vi "_CSM Message Communication Panel.vi"() -> ()   [LabVIEW 2017]
uses:
  _Support/Typedef/_CSM_GlobalLog_MSG.ctl
  _Support/Typedef/_CSM_Response Source Message.ctl
  _Support/Typedef/_CSM_GlobalLog_MSG_TYPE.ctl
  _Support/Priority Queue/Priority Queue.lvclass/Priority Queue.ctl
  _Polymophic/Add State(s) to Queue By BOOL(Element).vi
  _Polymophic/Build Synchronous Message with Arguments.vi
  _Polymophic/Build No-Reply Asynchronous Message with Arguments.vi
  AdvanceAPI/CSM - Keywords.vi
  AdvanceAPI/CSM - Convert Error to Argument.vi
  <vilib>/Utility/error.llb/Clear Errors.vi
  _Support/GlobalEvent/Gevt-ThreadQueueName.vi
  _Support/Common/Trim Single line Text.vi
  _Support/Process/CSMP-Sync Call.vi
  Utility/uuid.vi
  Utility/Build Error Cluster.vi
  Utility/Trim Both Whitespace.vi
  _Support/Process/CSMP-Async Call.vi
  _Support/CSMQ/_CSMObj-Message Check.vi
  _Support/CSMQ/_CSMObj-Enqueue Cross-Module Message.vi
  _Support/CSMQ/_CSMOFGV Get.vi
  _Support/Priority Queue/Enqueue Element.vi
  _Support/GlobalEvent/FGV-GlobalEventRef.vi
  <vilib>/Utility/config.llb/Read Key (String).vi
  <vilib>/Utility/config.llb/Write Key (String).vi
  _Support/FGV-BroadcastRegistry/global-CSMQ FGV Change Flag.vi
  _Support/CSMQ/_CSMOFGV.vi
  _Support/Error/CSM No Target Error.vi
  _Support/Error/CSM Not Allowed Message.vi
  _Support/Error/CSM Target Error.vi
  _Support/Error/CSM Unhandled State Error.vi
  _Support/Error/CSM Target Timeout Error.vi
  _Support/Message/Parse State with Arguments String.vi
  Communicable State Machine.lvlib
  <vilib>/Utility/config.llb/NI_LVConfig.lvlib
panel:
  in  "History":i32(listbox)
  in  "CSM 2":string(combo)
  in  "Refresh":bool
  in  "Arguments":string
  out "Response":string
  in  "Clear History":bool
  in  "History Length":i32=50 min=20 max=1000 step=1
  in  "CSM":string(combo)
  in  "Refresh CSM":bool
  in  "RespTMO(ms)":i32=10000 format="%.0p"
  in  "Sync (-@) 2":bool
  in  "Sync (-@)":bool
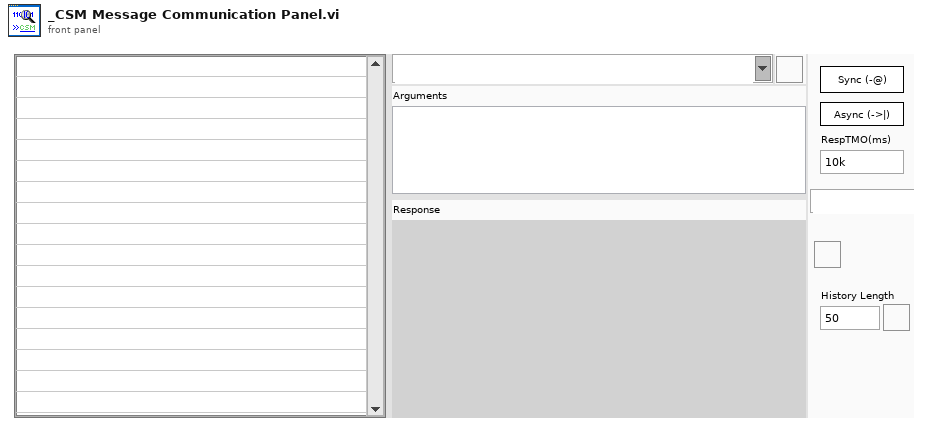
[diagram p1: front panel]
types:
  T1 = enum32{"Invalid", "Standard", "Closed", "Hidden", "Minimized", "Maximized"}
  T2 = enum32{"invalid app kind", "Development System", "Run Time System", "Student Edition", "Embedded LabVIEW", "Evaluation", "Custom"}
  T3 = cluster{"Shift":bool, "Ctrl":bool, "Alt":bool, "Cmd":bool, "Opt":bool}
  T4 = cluster{"Core":cluster{"Current VI Reference":refnum<vi>, "Close Panel on Exit?":bool}, "CSM Global Log Event":refnum<user-event>, "lvlps File":path, "MessageList":string[], "Toobar.advance":refnum<vi>[]}
  T5 = typedef "LVPoint32TypeDef.ctl" = cluster{"Horizontal":i32, "Vertical":i32}
  T6 = cluster{"Current VI Reference":refnum<vi>, "Close Panel on Exit?":bool}
  T7 = typedef "NI_LVConfig.lvlib/Config Data RefNum.ctl" = refnum<k1>
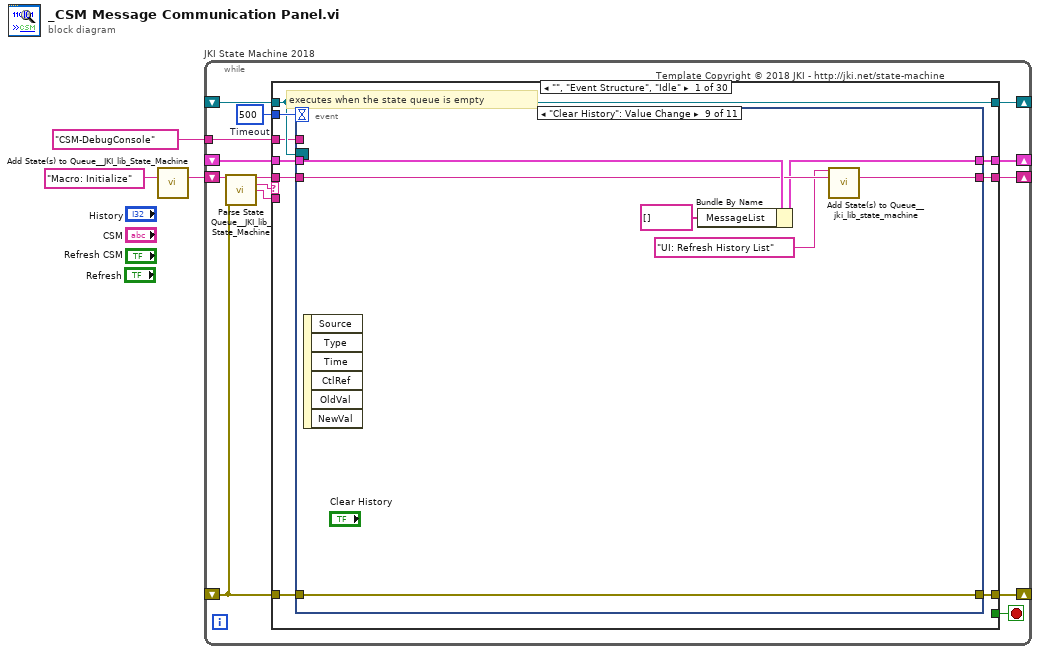
[diagram p0: block diagram]
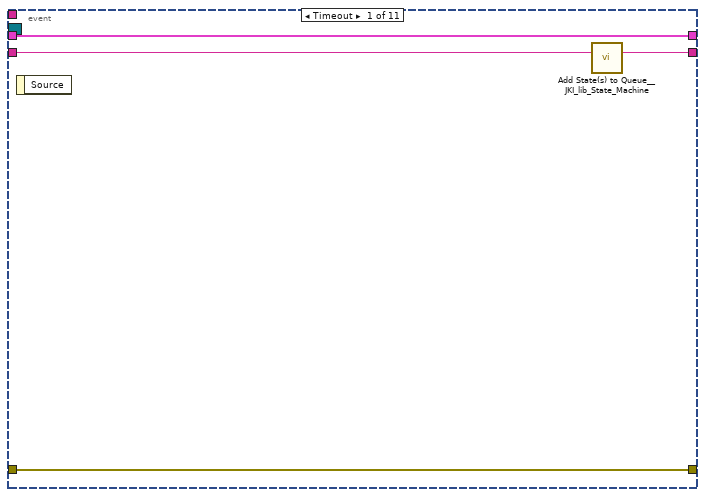
[diagram p2: hidden frame]
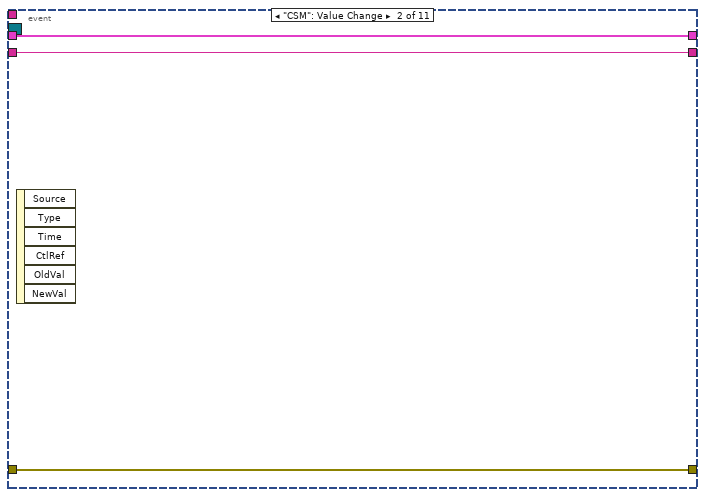
[diagram p3: hidden frame]
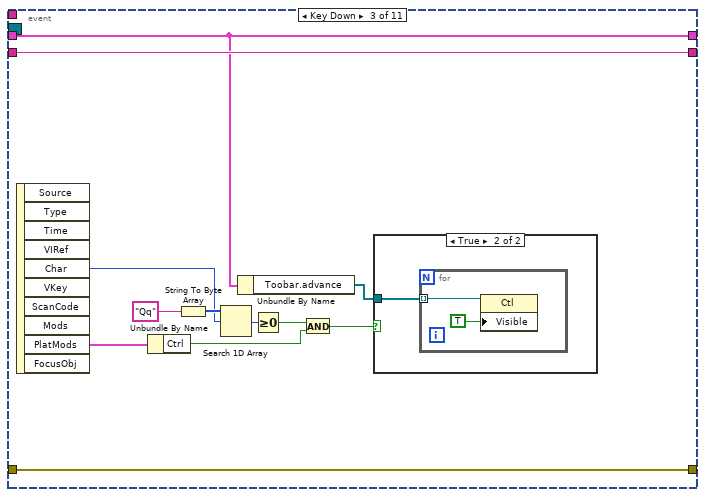
[diagram p4: hidden frame]
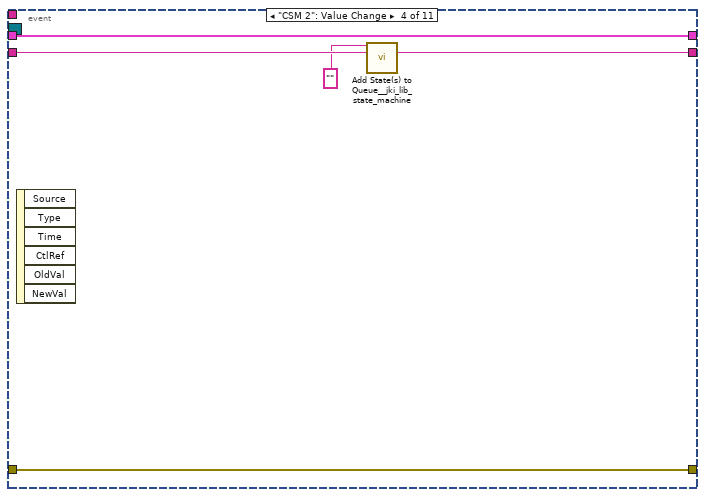
[diagram p6: hidden frame]
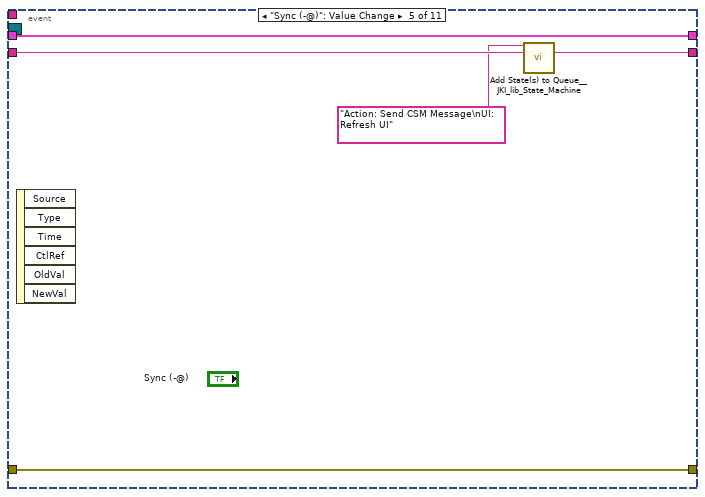
[diagram p7: hidden frame]
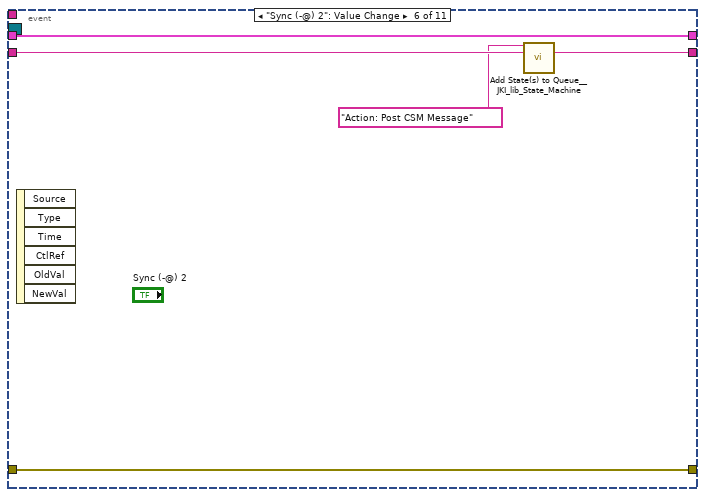
[diagram p8: hidden frame]
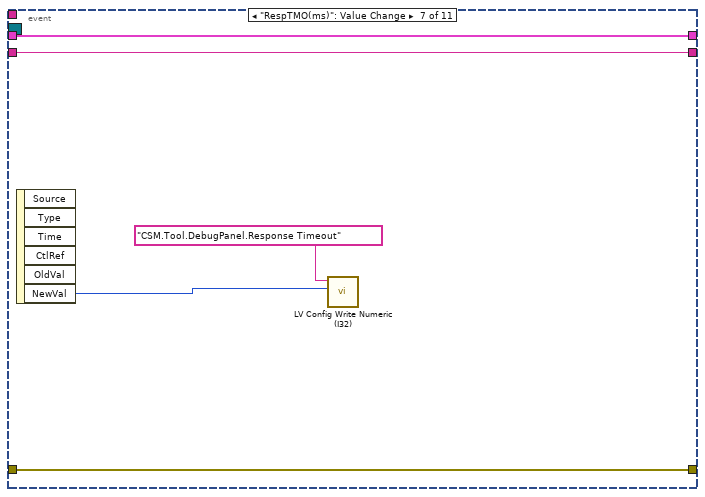
[diagram p9: hidden frame]
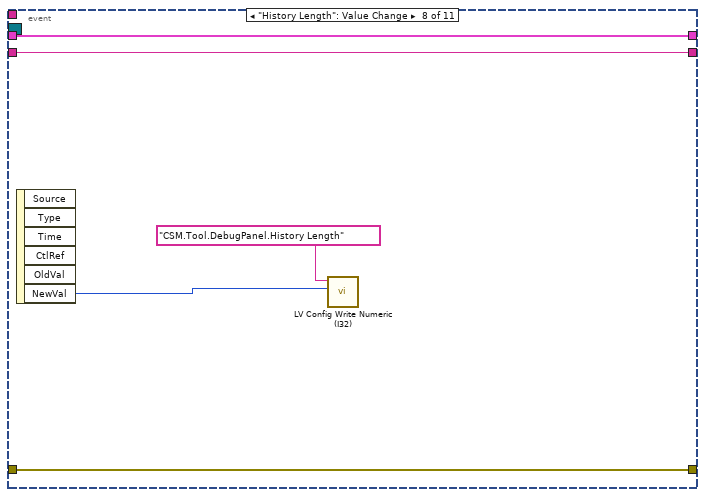
[diagram p10: hidden frame]
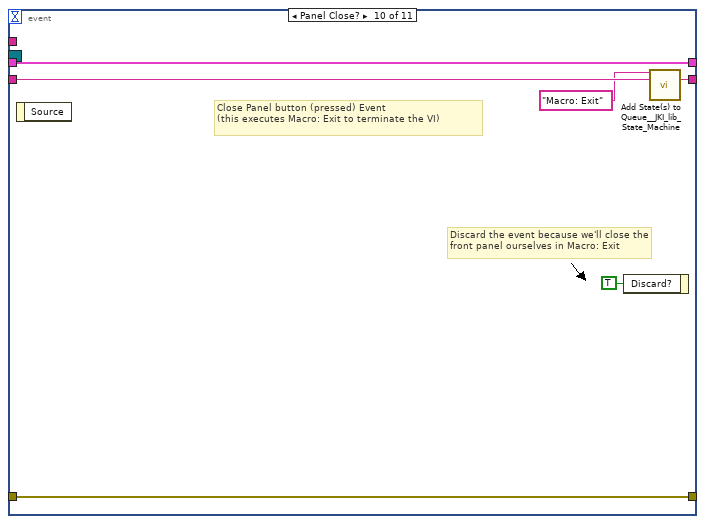
[diagram p11: hidden frame]
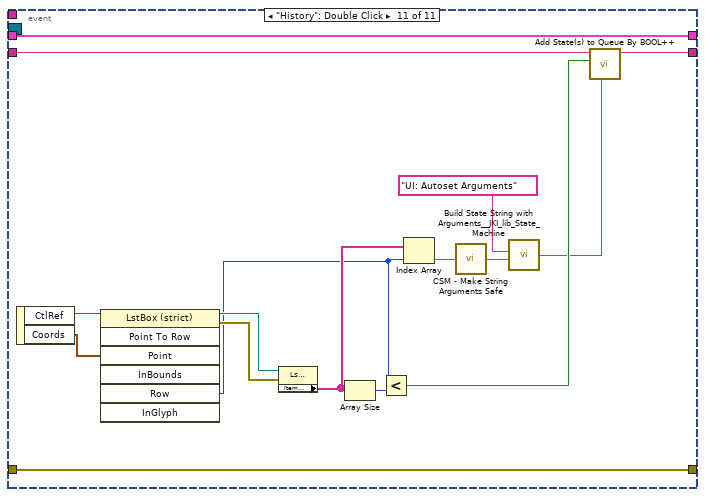
[diagram p12: hidden frame]
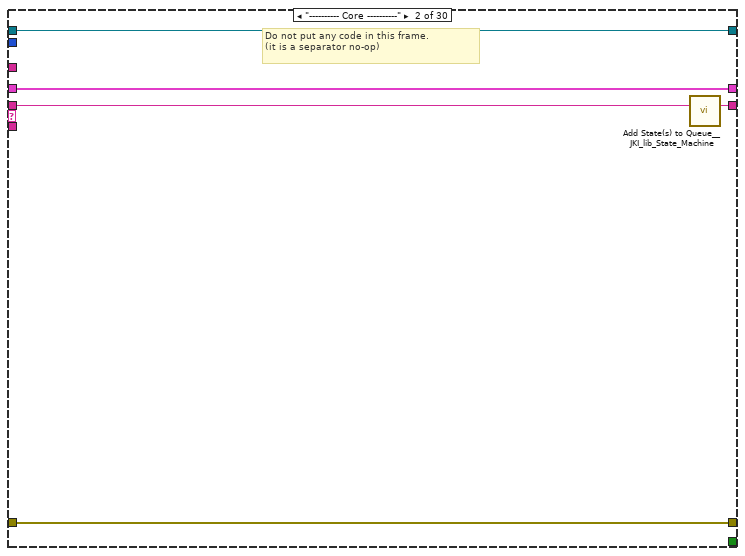
[diagram p13: hidden frame]
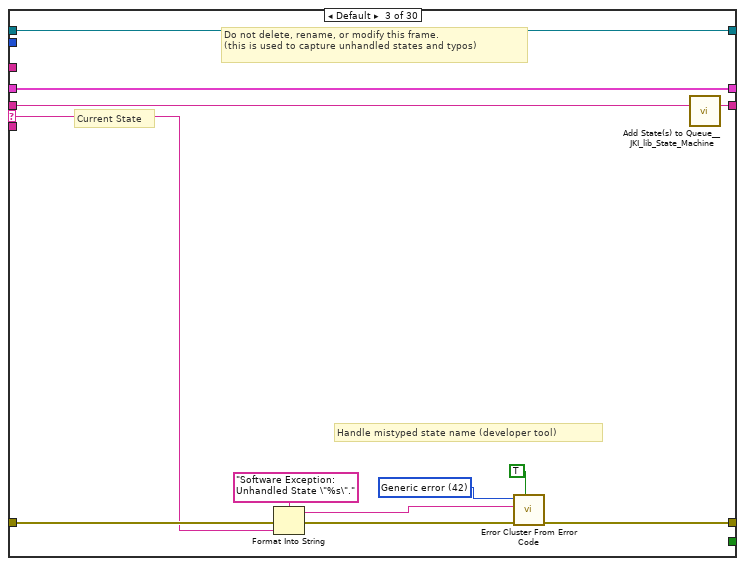
[diagram p14: hidden frame]
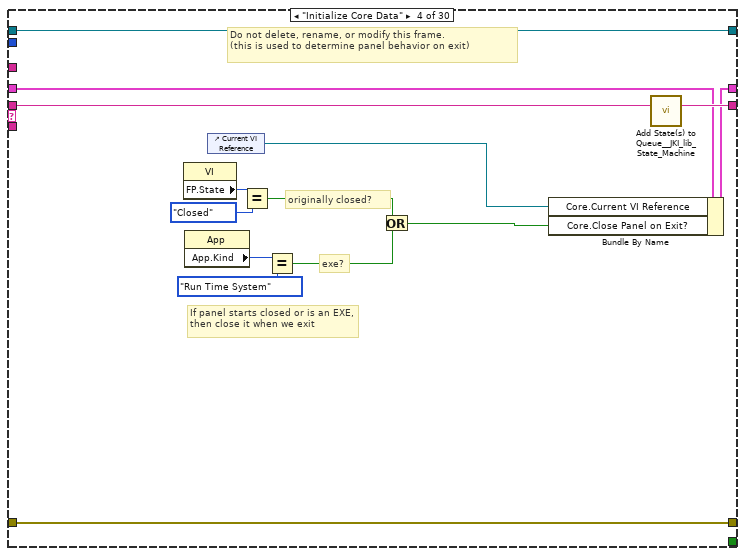
[diagram p15: hidden frame]
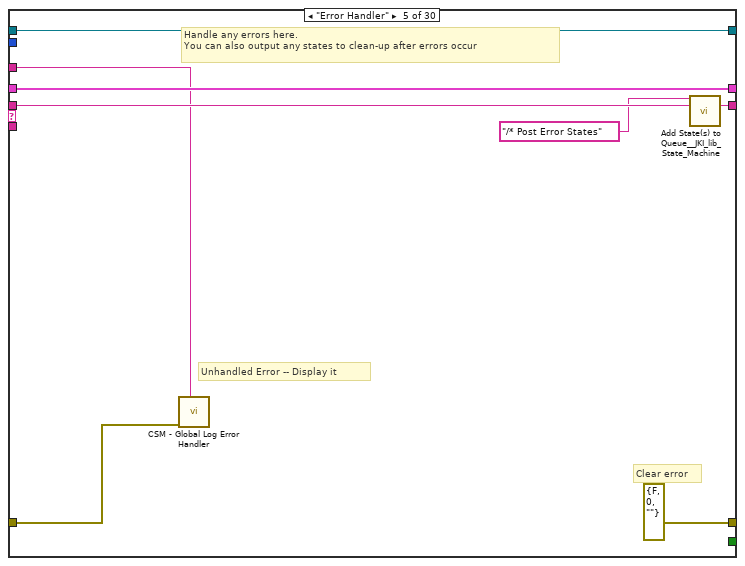
[diagram p16: hidden frame]
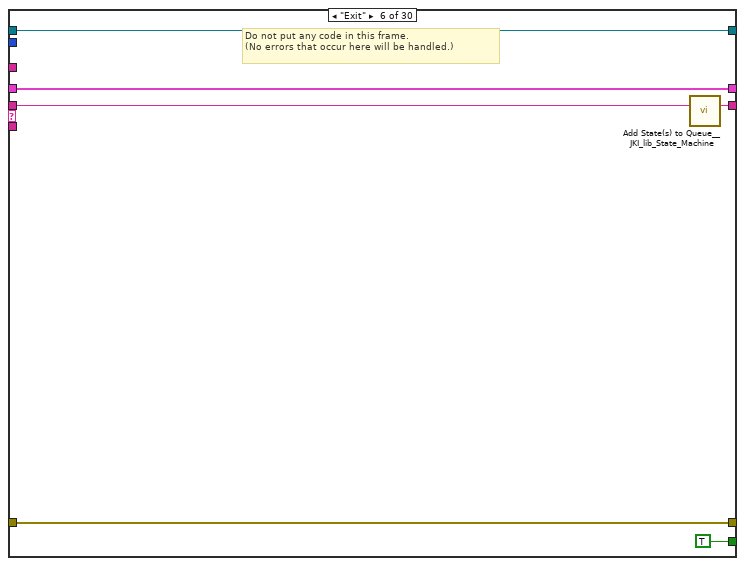
[diagram p17: hidden frame]
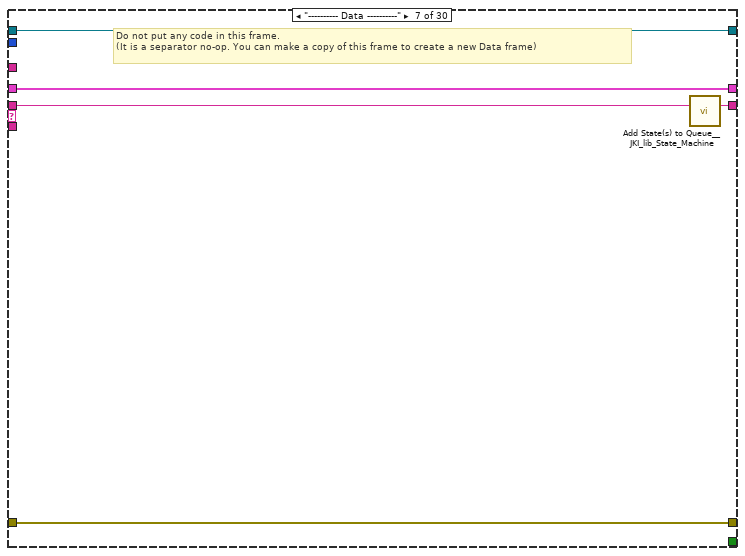
[diagram p18: hidden frame]
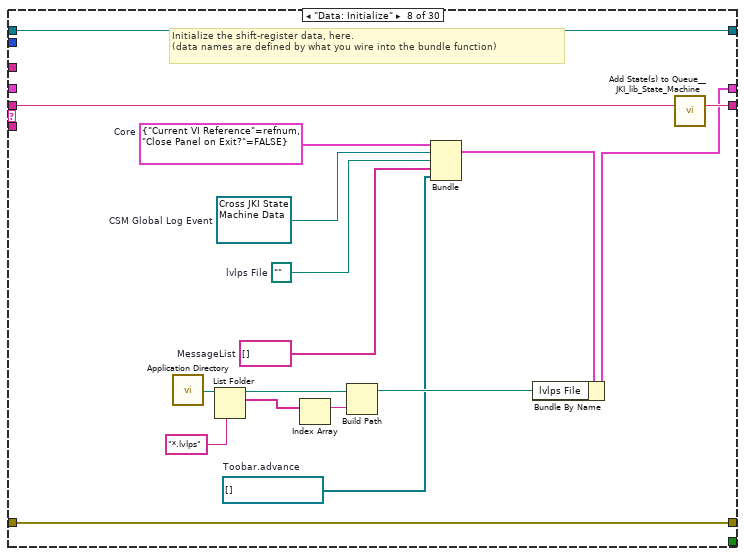
[diagram p19: hidden frame]
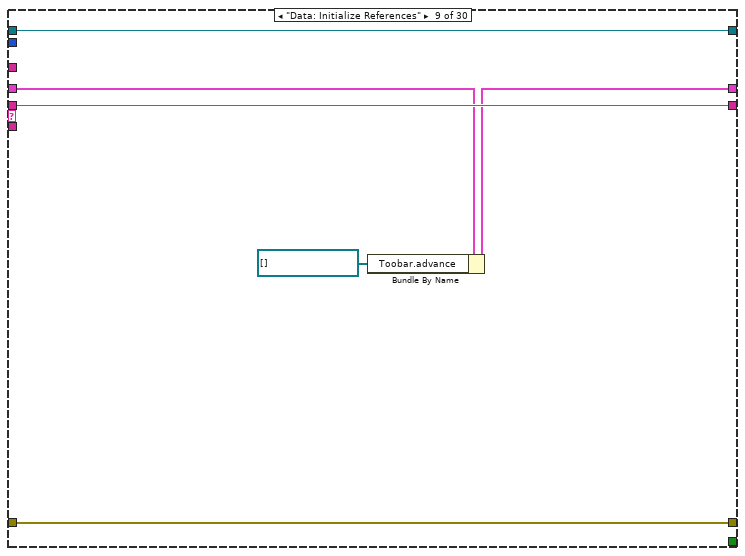
[diagram p20: hidden frame]
diagram:
  n1 = call <vilib>:"Add State(s) to Queue__JKI_lib_State_Machine.vi"("State(s) in (\"\")"="Macro: Initialize") -> ("States Out"=w2:string)  [unwired: 14 in]
  n2 = while "JKI State Machine 2018" {
    shift-right: [w10] -> _
    shift-left: _ -> [w9]
    shift-right: [w13] -> _
    shift-left: _ -> [w7]
    shift-right: [w12] -> _
    shift-left: w2 -> [w14]
    shift-right: [w6] -> _
    shift-left: _ -> [w5]
    tunnel: "CSM-DebugConsole" -> [w4]
    stop <- w11 stop-if-true
    w8 = 500  # Timeout
    # "Template Copyright © 2018 JKI - http://jki.net/state-machine"
    n3 = call <vilib>:"Parse State Queue__JKI_lib_State_Machine.vi"("State Queue"=w14, "Error In (no error)"=w7) -> ("Remaining States"=w16:string, "Current State"=w17:string, "Arguments"=w15:string)  [unwired: 11 in]
    n4 = case shown="\"\", \"Event Structure\", \"Idle\"" w17 {
      selector: w17 -> [_ _ w109 _ _ _ _ _ _ _ _ _ _ _ _ _ _ _ _ _ _ _ _ _ _ _ _ _ _ _]
      tunnel: w16 -> [w26 w107 w113 w133 w141 w147 w152 w169 w174 w186 w217 w248 w264 w269 w276 w283 w288 w300 w310 w322 w401 w412 w425 w429 w435 w441 w452 w457 w467 w489]
      tunnel: w15 -> [_ _ _ _ _ _ _ _ _ _ _ w243 _ _ _ _ _ _ w305 w316 w399 _ _ _ _ _ _ _ _ _]
      tunnel: w9 -> [w24 w104 w111 w126 w138 w145 w149 _ w173 w179 w210 w245 w259 w266 w274 w279 w285 w296 w308 w318 w396 w410 w424 w427 w432 w438 w449 w454 w465 w487]
      tunnel: [w23 w105 w115 w130 errorcluster {"status"=FALSE, "code"=0, "source"=""} ("error out") w144 w150 w166 w175 w178 w211 w246 w260 w267 w272 w280 w286 w298 w306 w319 w402 w413 w426 w430 w433 w439 w450 w455 w461 w485] -> w13
      tunnel: w7 -> [w22 w105 w114 w130 w137 w144 w150 w166 w175 _ _ w246 w261 w267 _ _ w286 w298 w307 w320 w402 w413 w426 w430 w433 w439 w450 w455 _ _]
      tunnel: [w25 w106 w112 w132 w140 w146 w151 w168 w174 w186 w217 w248 w263 w268 w275 w282 w287 w299 w309 w321 w401 w412 w425 w429 w434 w440 w451 w456 w466 w488] -> w12
      tunnel: [_ _ _ _ _ TRUE _ _ _ _ _ _ _ _ _ _ _ _ _ _ _ _ _ _ _ _ _ _ _ _] -> w11
      tunnel: [w21 w104 w111 w131 w138 w145 w149 w161 w171 w184 w210 w239 w259 w266 w274 w279 w285 w296 w308 w318 w396 w410 w424 w427 w432 w438 w449 w454 w465 w487] -> w10
      tunnel: w8 -> [w20 _ _ _ _ _ _ _ _ _ _ _ _ _ _ _ _ _ _ _ _ _ _ _ _ _ _ _ _ _]
      tunnel: [w19 w103 w108 w120 w135 w142 w148 w164 w172 w185 w216 w247 w258 w265 w273 w281 w284 w297 w304 w315 w400 w411 w423 w428 w431 w436 w442 w453 w464 w486] -> w6
      tunnel: w5 -> [w19 w103 w108 w120 w135 w142 w148 w164 w172 w185 w216 w247 w258 w265 _ w281 w284 w297 w304 w315 w400 w411 w423 w428 w431 w436 w442 w453 w464 w486]
      tunnel: w4 -> [w18 _ _ _ w134 _ _ _ _ w176 w208 _ _ _ _ _ _ _ _ _ _ _ _ _ _ _ _ _ _ _]
      frame "", "Event Structure", "Idle" {
        # "executes when the state queue is empty"
        n5 = event shown="[8] \"Clear History\": Value Change" {
          selector: w19 -> [_ _ _ _ _ _ _ _ _ _ _]
          dyn-events: _ -> [_ _ _ _ _ _ _ _ _ _ _]
          timeout: w20 -> [_ _ _ _ _ _ _ _ _ _ _]
          tunnel: w26 -> [w30 w33 w45 w50 w55 w60 w68 w73 w77 w86 w94]
          tunnel: [w29 w33 w45 w51 w56 w61 w68 w73 w78 w85 w95] -> w25
          tunnel: w24 -> [w27 w31 w34 w52 w57 w62 w66 w71 w79 w83 w101]
          tunnel: [w28 w32 w44 w53 w58 w63 w67 w72 w80 w84 w102] -> w23
          tunnel: w22 -> [w28 w32 w44 w53 w58 w63 w67 w72 w80 w84 w102]
          tunnel: [w27 w31 w34 w52 w57 w62 w66 w71 w75 w83 w101] -> w21
          tunnel: w18 -> [_ _ _ _ _ _ _ _ _ _ _]
          event Timeout {
            n6 = event-data() -> ()  [unwired: 1 in, 1 out]
            n7 = call <vilib>:"Add State(s) to Queue__JKI_lib_State_Machine.vi"("State(s) in (\"\")"=w30) -> ("States Out"=w29:string)  [unwired: 14 in]
          }
          event "CSM": Value Change {
            n8 = event-data() -> ()  [unwired: 1 in, 6 out]
          }
          event Key Down {
            n9 = event-data() -> ("Char"=w35:i16, "PlatMods"=w36:T3)  [unwired: 1 in, 8 out]
            n10 = Unbundle By Name(w36) -> ("Ctrl"=w39:bool)
            n11 = String To Byte Array(string="Qq") -> (unsigned byte array=w41:u8[])
            n12 = Search 1D Array(1D array=w41, element=w35) -> (index of element=w42:i32)  [unwired: 1 in]
            n13 = Unbundle By Name(w34) -> ("Toobar.advance"=w37:refnum<vi>[])
            n14 = Greater Or Equal To 0?(x=w42) -> (x >= 0?=w43:bool)
            n15 = And(x=w43, y=w39) -> (x .and. y?=w38:bool)
            n16 = case shown="True" w38 {
              tunnel: w37 -> [_ w46]
              frame False {
              }
              frame True {
                n17 = for {
                  tunnel: w46 -> [w48] mode=indexing
                  n18 = property class="Ctl"(reference=w48, "Visible"=TRUE) -> ()  [unwired: 1 in, 2 out]
                }
              }
            }
          }
          event "CSM 2": Value Change {
            n19 = event-data() -> ()  [unwired: 1 in, 6 out]
            n20 = call <vilib>:"Add State(s) to Queue__jki_lib_state_machine.vi"("State(s) in Front (\"\")"="" ("State(s) in Front (\"\")"), "State(s) in (\"\")"=w50) -> ("States Out"=w51:string)  [unwired: 13 in]
          }
          event "Sync (-@)": Value Change {
            n21 = event-data() -> ()  [unwired: 1 in, 6 out]
            n22 = call <vilib>:"Add State(s) to Queue__JKI_lib_State_Machine.vi"("State(s) in Front (\"\")"="Action: Send CSM Message\nUI: Refresh UI" ("State(s) in Front (\"\")"), "State(s) in (\"\")"=w55) -> ("States Out"=w56:string)  [unwired: 13 in]
          }
          event "Sync (-@) 2": Value Change {
            n23 = event-data() -> ()  [unwired: 1 in, 6 out]
            n24 = call <vilib>:"Add State(s) to Queue__JKI_lib_State_Machine.vi"("State(s) in Front (\"\")"="Action: Post CSM Message" ("State(s) in Front (\"\")"), "State(s) in (\"\")"=w60) -> ("States Out"=w61:string)  [unwired: 13 in]
          }
          event "RespTMO(ms)": Value Change {
            n25 = event-data() -> ("NewVal"=w64:i32)  [unwired: 1 in, 5 out]
            n26 = call <resource>:"LV Config Write Numeric (I32).vi"("value"=w64, "key"="CSM.Tool.DebugPanel.Response Timeout") -> ()  [unwired: 5 in, 1 out]
          }
          event "History Length": Value Change {
            n27 = event-data() -> ("NewVal"=w69:i32)  [unwired: 1 in, 5 out]
            n28 = call <resource>:"LV Config Write Numeric (I32).vi"("value"=w69, "key"="CSM.Tool.DebugPanel.History Length") -> ()  [unwired: 5 in, 1 out]
          }
          event "Clear History": Value Change {
            n29 = event-data() -> ()  [unwired: 1 in, 6 out]
            n30 = Bundle By Name(cluster=w79, "MessageList"=string[] []) -> (w75:T4)
            n31 = call <vilib>:"Add State(s) to Queue__jki_lib_state_machine.vi"("State(s) in Front (\"\")"="UI: Refresh History List" ("State(s) in Front (\"\")"), "State(s) in (\"\")"=w77) -> ("States Out"=w78:string)  [unwired: 13 in]
          }
          event Panel Close? {
            # "Discard the event because we'll close the front panel ourselves in Macro: Exit"
            # "Close Panel button (pressed) Event\n(this executes Macro: Exit to terminate the VI)"
            n32 = event-data() -> ()  [unwired: 1 in, 1 out]
            n33 = event-data("Discard?"=TRUE) -> ()  [unwired: 1 in, 1 out]
            n34 = call <vilib>:"Add State(s) to Queue__JKI_lib_State_Machine.vi"("State(s) in Front (\"\")"="Macro: Exit", "State(s) in (\"\")"=w86) -> ("States Out"=w85:string)  [unwired: 13 in]
          }
          event "History": Double Click {
            n35 = event-data() -> ("CtlRef"=w100:refnum<vi>, "Coords"=w88:T5)  [unwired: 1 in]
            n36 = invoke class="LstBox (strict)" method="Point To Row"(reference=w100, "Point"=w88) -> (reference out=w99:refnum<vi>, error out=w98:errorcluster, "Row"=w87:i32)  [unwired: 5 in, 4 out]
            n37 = property class="LstBox (strict)"(reference=w99, error in=w98) -> ("Item Names"=w96:string[])  [unwired: 2 out]
            n38 = Array Size(array=w96) -> (size(s)=w97:i32)
            n39 = Less?(x=w87, y=w97) -> (x < y?=w93:bool)
            n40 = Index Array(array=w96, index=w87) -> (element=w92:string)
            n41 = call "CSM - Make String Arguments Safe.vi"("Argurment String"=w92) -> ("Safe Argurment String"=w91:string)  [unwired: 8 in]
            n42 = call <vilib>:"Build State String with Arguments__JKI_lib_State_Machine.vi"("Arguments (\"\")"=w91, "State"="UI: Autoset Arguments") -> ("State with Arguments"=w89:string)  [unwired: 4 in]
            n43 = call-poly "Add State(s) to Queue By BOOL++.vi"("TRUE(\"\")"=w89, "Condition"=w93, "State Queue(\"\")"=w94) -> ("Remaining States"=w95:string)  [unwired: 8 in]
          }
        }
      }
      frame "---------- Core ----------" {
        # "Do not put any code in this frame.\n(it is a separator no-op)"
        n44 = call <vilib>:"Add State(s) to Queue__JKI_lib_State_Machine.vi"("State(s) in (\"\")"=w107) -> ("States Out"=w106:string)  [unwired: 14 in]
      }
      frame Default {
        w118 = 42 items=["No error", "Argument error", "Memory is full", "Out of zone", "End of file", "File already open", "Generic file I/O error", "File not found", "File permission error", "Disk is full", "Duplicate path", "Too many files open", "System feature not enabled", "Resource file not found", "Cannot add resource", "Resource not found", "Image not found", "Image memory error", "Pen does not exist", "Config type invalid", "Config token not found", "Config parse error", "Config memory error", "Bad external code format", "Bad external code offset", "External code not present", "Null window", "Destroy window error", "Null menu", "Print aborted", "Bad print record", "Print driver error", "Windows error during printing", "Memory error during printing", "Print dialog error", "Generic print error", "Invalid device refnum", "Device not found", "Device parameter error", "Device unit error", "Cannot open device", "Device call aborted", "Generic error", "Cancelled by user", "Object ID too low", "Object ID too high", "Object not in heap", "Unknown heap", "Unknown object (invalid DefProc)", "Unknown object (DefProc not in table)", "Message out of range", "Invalid (null) method", "Unknown message", "Manager call not supported", "Bad address", "Network operation in progress", "Network operation timed out", "Connection is busy", "Network attribute not supported", "Network error", "Address in use", "System out of memory", "Connection aborted", "Connection refused", "Not connected", "Already connected", "Connection closed", "Initialization error (interapplication manager)", "Bad occurrence", "Wait on unbound occurrence handler", "Occurrence queue overflow", "Datalog type conflict", "Unused", "Unrecognized type (interapplication manager)", "Memory corrupt", "Failed to make temporary DLL", "Old CIN version", "Drag socket not found", "Failed to load drop-object", "Failed to register OLE object", "Failed to release OLE object", "Format specifier type mismatch", "Unknown format specifier", "Too few format specifiers", "Too many format specifiers", "Scan failed", "Newer CIN version", "Error converting to variant", "Runtime menu error", "Password tampered", "Variant attribute not found", "Incompatible variant data type", "Event data is not available", "Event Store is not present", "Occurrence is not found", "Event Queue is not created", "Event info is not available", "Refnum passed is NULL", "Error retrieving Class GUID", "Error retrieving CoClass GUID", "Error retrieving TypeLib GUID.", "Bad built application magic bytes.", "Specific driver is different from the specific driver associated with the Logical Name.", "There is no session opened to the class driver.", "Max Error", "MAX - Error with config objects", "MAX - Error loading configuration", "MAX - Group not supported"]
        # "Current State"
        # "Do not delete, rename, or modify this frame.\n(this is used to capture unhandled states and typos)"
        # "Handle mistyped state name (developer tool)"
        n45 = Format Into String(format string="Software Exception: Unhandled State \"%s\"." ("message"), error in=w114, w109) -> (resulting string=w117:string, error out=w116:errorcluster)  [unwired: 1 in]
        n46 = call <vilib>:"Error Cluster From Error Code.vi"("show call chain? (False)"=TRUE, "error in (no error)"=w116, "error message (\"\")"=w117, "error code (0)"=w118) -> ("error out"=w115:errorcluster)  [unwired: 5 in]
        n47 = call <vilib>:"Add State(s) to Queue__JKI_lib_State_Machine.vi"("State(s) in (\"\")"=w113) -> ("States Out"=w112:string)  [unwired: 14 in]
      }
      frame "Initialize Core Data" {
        # "Do not delete, rename, or modify this frame.\n(this is used to determine panel behavior on exit)"
        # "originally closed?"
        # "exe?"
        # "If panel starts closed or is an EXE, then close it when we exit"
        n48 = property class="VI"() -> ("FP.State"=w123:T1)  [unwired: 2 in, 2 out]
        n49 = property class="App"() -> ("App.Kind"=w129:T2)  [unwired: 2 in, 2 out]
        n50 = control-ref of="Current VI Reference"() -> (w124:refnum<vi>)
        n51 = Equal?(x=w123, y=T1."Closed" ("Front Panel Window:State")) -> (x = y?=w121:bool)
        n52 = Equal?(x=w129, y=T2."Run Time System" ("Application:Kind")) -> (x = y?=w127:bool)
        n53 = Or(x=w121, y=w127) -> (x .or. y?=w125:bool)
        n54 = Bundle By Name(cluster=w126, "Core.Current VI Reference"=w124, "Core.Close Panel on Exit?"=w125) -> (w131:T4)
        n55 = call <vilib>:"Add State(s) to Queue__JKI_lib_State_Machine.vi"("State(s) in (\"\")"=w133) -> ("States Out"=w132:string)  [unwired: 14 in]
      }
      frame "Error Handler" {
        # "Unhandled Error -- Display it"
        # "Handle any errors here.\nYou can also output any states to clean-up after errors occur"
        # "Clear error"
        n56 = call "CSM - Global Log Error Handler.vi"("Place(\"\" to use VI's Name)"=w134, "Error in"=w137) -> ()  [unwired: 9 in, 1 out]
        n57 = call <vilib>:"Add State(s) to Queue__JKI_lib_State_Machine.vi"("State(s) in Front (\"\")"="/* Post Error States", "State(s) in (\"\")"=w141) -> ("States Out"=w140:string)  [unwired: 13 in]
      }
      frame "Exit" {
        # "Do not put any code in this frame.\n(No errors that occur here will be handled.)"
        n58 = call <vilib>:"Add State(s) to Queue__JKI_lib_State_Machine.vi"("State(s) in (\"\")"=w147) -> ("States Out"=w146:string)  [unwired: 14 in]
      }
      frame "---------- Data ----------" {
        # "Do not put any code in this frame.\n(It is a separator no-op. You can make a copy of this frame to create a new Data frame)"
        n59 = call <vilib>:"Add State(s) to Queue__JKI_lib_State_Machine.vi"("State(s) in (\"\")"=w152) -> ("States Out"=w151:string)  [unwired: 14 in]
      }
      frame "Data: Initialize" {
        w153 = refnum<vi>[] []  # Toobar.advance
        w160 = string[] []  # MessageList
        w162 = path ""  # lvlps File
        w163 = refnum<user-event> refnum  # CSM Global Log Event
        w165 = T6 {"Current VI Reference"=refnum, "Close Panel on Exit?"=FALSE}  # Core
        # "Initialize the shift-register data, here.\n(data names are defined by what you wire into the bundle function)"
        n60 = call <vilib>:"Application Directory.vi"() -> ("Application Directory"=w158:path)
        n61 = List Folder(path=w158, pattern="*.lvlps" ("pattern(ini by default)")) -> (path out=w157:path, filenames=w156:string[])  [unwired: 2 in, 2 out]
        n62 = Index Array(array=w156) -> (element=w154:string)  [unwired: 1 in]
        n63 = Build Path(base path=w157, name or relative path=w154) -> (appended path=w155:path)
        n64 = Bundle("Core"=w165, "CSM Global Log Event"=w163, "lvlps File"=w162, "MessageList"=w160, "Toobar.advance"=w153) -> (w167:T4)  [unwired: 1 in]
        n65 = Bundle By Name(cluster=w167, "lvlps File"=w155) -> (w161:T4)
        n66 = call <vilib>:"Add State(s) to Queue__JKI_lib_State_Machine.vi"("State(s) in (\"\")"=w169) -> ("States Out"=w168:string)  [unwired: 14 in]
      }
      frame "Data: Initialize References" {
        n67 = Bundle By Name(cluster=w173, "Toobar.advance"=refnum<vi>[] []) -> (w171:T4)
      }
      frame "Data: Load Arguments Config File" {
        n68 = Unbundle By Name(w179) -> ("lvlps File"=w183:path)
        n69 = call <vilib>:"Check if File or Folder Exists.vi"("path"=w183) -> ("error out"=w180:errorcluster, "file or folder exists?"=w181:bool, "dup path"=w182:path)  [unwired: 8 in]
        n70 = case shown="True" w181 {
          tunnel: [w187 w198] -> w178
          tunnel: w182 -> [_ w197]
          tunnel: w180 -> [w187 w196]
          tunnel: [_ w188] -> w177
          tunnel: w176 -> [_ w189]
          frame False {
          }
          frame True {
            n71 = call <vilib>:"Open Config Data.vi"("error in (no error)"=w196, "configuration file path"=w197) -> ("error out"=w195:errorcluster, "refnum"=w191:T7)  [unwired: 7 in, 1 out]
            n72 = call <vilib>:"Get Key Names.vi"("section"=w189, "error in (no error)"=w195, "refnum"=w191) -> ("error out"=w193:errorcluster, "key names"=w192:string[], "refnum out"=w194:T7)  [unwired: 5 in, 1 out]
            n73 = for {
              shift-right: [w205] -> w199
              shift-left: w193 -> [w207]
              shift-right: [w206] -> w190
              shift-left: w194 -> [w201]
              tunnel: w189 -> [w204]
              tunnel: w192 -> [w203] mode=indexing
              tunnel: [w200] -> w188 mode=indexing
              n74 = call-poly <vilib>:"Read Key.vi"("section"=w204, "error in (no error)"=w207, "default value"="" ("Value"), "key"=w203, "refnum"=w201) -> ("error out"=w205:errorcluster, "value"=w200:string, "refnum out"=w206:T7)  [unwired: 3 in, 1 out]
            }
            n75 = call <vilib>:"Close Config Data.vi"("error in (no error)"=w199, "refnum"=w190) -> ("error out"=w198:errorcluster)  [unwired: 8 in, 1 out]
          }
        }
        n76 = Bundle By Name(cluster=w179, "MessageList"=w177) -> (w184:T4)
      }
      frame "Data: Save Arguments Config File" {
        n77 = Unbundle By Name(w210) -> ("MessageList"=w209:string[], "lvlps File"=w215:path)
        n78 = call <vilib>:"Check if File or Folder Exists.vi"("path"=w215) -> ("error out"=w212:errorcluster, "file or folder exists?"=w213:bool, "dup path"=w214:path)  [unwired: 8 in]
        n79 = case shown="True" w213 {
          tunnel: [w218 w224] -> w211
          tunnel: w214 -> [_ w223]
          tunnel: w212 -> [w218 w222]
          tunnel: w209 -> [_ w221]
          tunnel: w208 -> [_ w219]
          frame False {
          }
          frame True {
            n80 = call <vilib>:"Open Config Data.vi"("error in (no error)"=w222, "configuration file path"=w223) -> ("error out"=w227:errorcluster, "refnum"=w226:T7)  [unwired: 7 in, 1 out]
            n81 = for {
              shift-right: [w234] -> w225
              shift-left: w227 -> [w235]
              shift-right: [w232] -> w220
              shift-left: w226 -> [w233]
              tunnel: w221 -> [w230] mode=indexing
              tunnel: w219 -> [w231]
              i -> [w229]
              n82 = Format Into String(w229) -> (resulting string=w228:string)  [unwired: 3 in, 1 out]
              n83 = call-poly <vilib>:"Write Key.vi"("section"=w231, "error in (no error)"=w235, "value"=w230, "key"=w228, "refnum"=w233) -> ("error out"=w234:errorcluster, "refnum out"=w232:T7)  [unwired: 4 in, 1 out]
            }
            n84 = call <vilib>:"Close Config Data.vi"("error in (no error)"=w225, "refnum"=w220) -> ("error out"=w224:errorcluster)  [unwired: 8 in, 1 out]
          }
        }
      }
      frame "Data: Update Message List" {
        n85 = Unbundle By Name(w245) -> ("MessageList"=w244:string[])
        n86 = call "CSM - Revert Arguments-Safe String.vi"("Safe Argurment String"=w243) -> ("Origin Argurment String"=w242:string)  [unwired: 8 in]
        n87 = Build Array (concatenate)(w242, w244) -> (w241:string[])
        n88 = for {
          tunnel: w241 -> [w252] mode=indexing
          shift-right: [w251] -> w237
          shift-left: string[] [] -> [w250]
          i -> [w249]
          n89 = Search 1D Array(1D array=w250, element=w252) -> (index of element=w253:i32)  [unwired: 1 in]
          n90 = case shown="-1" w253 {
            tunnel: w252 -> [_ w257]
            tunnel: [w254 w255] -> w251
            tunnel: w250 -> [w254 w256]
            tunnel: w249 -> [_ _]
            frame Default {
            }
            frame -1 {
              n91 = Build Array (concatenate)(w256, w257) -> (w255:string[])
            }
          }
        }
        n92 = Array Subset(array=w237, length="History Length") -> (w238:string[])  [unwired: 1 in]
        n93 = Bundle By Name(cluster=w245, "MessageList"=w238) -> (w239:T4)
      }
      frame "Data: Cleanup" {
        # "Cleanup any data and references, here.\n(this is called automatically, by the Macro: Exit)"
        n94 = Unbundle By Name(w259) -> ("Core.Current VI Reference"=w262:refnum<vi>)
        n95 = Close Reference(reference=w262, error in (no error)=w261) -> (error out=w260:errorcluster)
        n96 = call <vilib>:"Add State(s) to Queue__JKI_lib_State_Machine.vi"("State(s) in (\"\")"=w264) -> ("States Out"=w263:string)  [unwired: 14 in]
      }
      frame "---------- Events ----------" {
        # "Do not put any code in this frame.\n(It is a separator no-op. You can make a copy of this frame to create a new UI frame)"
        n97 = call <vilib>:"Add State(s) to Queue__JKI_lib_State_Machine.vi"("State(s) in (\"\")"=w269) -> ("States Out"=w268:string)  [unwired: 14 in]
      }
      frame "Events: Register" {
        # "Do not put any code in this frame.\n(It is a separator no-op. You can make a copy of this frame to create a new UI frame)"
        n98 = call "CSM - Global Log Event.vi"() -> ("Error out"=w270:errorcluster, "CSM Global Log Event"=w271:refnum<user-event>)  [unwired: 10 in]
        n99 = register-events(error in=w270, w271) -> (reference out=w273:refnum<event-registration>, error out=w272:errorcluster)  [unwired: 1 in]
        n100 = call <vilib>:"Add State(s) to Queue__JKI_lib_State_Machine.vi"("State(s) in (\"\")"=w276) -> ("States Out"=w275:string)  [unwired: 14 in]
      }
      frame "Events: Unregister" {
        # "Do not put any code in this frame.\n(It is a separator no-op. You can make a copy of this frame to create a new UI frame)"
        n101 = Unbundle By Name(w279) -> ("CSM Global Log Event"=w278:refnum<user-event>)
        n102 = call "CSM - Destroy Global Log Event.vi"("CSM Global Log Event"=w278) -> ("Error out"=w277:errorcluster)  [unwired: 10 in]
        n103 = Unregister For Events(event registration refnum=w281, error in=w277) -> (error out=w280:errorcluster)
        n104 = call <vilib>:"Add State(s) to Queue__JKI_lib_State_Machine.vi"("State(s) in (\"\")"=w283) -> ("States Out"=w282:string)  [unwired: 14 in]
      }
      frame "---------- UI ----------" {
        # "Do not put any code in this frame.\n(It is a separator no-op. You can make a copy of this frame to create a new UI frame)"
        n105 = call <vilib>:"Add State(s) to Queue__JKI_lib_State_Machine.vi"("State(s) in (\"\")"=w288) -> ("States Out"=w287:string)  [unwired: 14 in]
      }
      frame "UI: Initialize" {
        # "Initialize the User Interface, here.\n(this is called automatically, by the Macro: Init)"
        n106 = Unbundle By Name(w296) -> ("Toobar.advance"=w295:refnum<vi>[])
        n107 = call <resource>:"LV Config Read Numeric (I32).vi"("default value"=50, "key"="CSM.Tool.DebugPanel.History Length") -> ("value"=w291:i32)  [unwired: 3 in, 2 out]
        n108 = call <resource>:"LV Config Read Numeric (I32).vi"("default value"=30000, "key"="CSM.Tool.DebugPanel.Response Timeout") -> ("value"=w292:i32)  [unwired: 3 in, 2 out]
        n109 = disable-structure shown="Disabled" {
          disable-tunnel: w295 -> [w301 _]
          frame Disabled {
            n110 = for {
              tunnel: w301 -> [w303] mode=indexing
              n111 = property class="Ctl"(reference=w303, "Visible"=FALSE) -> ()  [unwired: 1 in, 2 out]
            }
          }
          frame Enabled {
          }
        }
        n112 = local write "History Length"(w291) -> ()
        n113 = local write "RespTMO(ms)"(w292) -> ()
        n114 = call <vilib>:"Add State(s) to Queue__JKI_lib_State_Machine.vi"("State(s) in (\"\")"=w300) -> ("States Out"=w299:string)  [unwired: 14 in]
      }
      frame "UI: Cursor Set" {
        # "Argument"
        # "Set and Unset Cursor Busy.\n(Usage: \"UI: Cursor Set >> Busy|Idle\")"
        n115 = case shown="\"Idle\", Default" w305 {
          tunnel: w307 -> [w312 w314]
          tunnel: [w311 w313] -> w306
          frame "Idle", Default {
            n116 = call <vilib>:"Unset Busy.vi"("error in (no error)"=w312) -> ("error out"=w311:errorcluster)  [unwired: 10 in]
          }
          frame "Busy" {
            n117 = call <vilib>:"Set Busy.vi"("error in (no error)"=w314) -> ("error out"=w313:errorcluster)  [unwired: 9 in, 1 out]
          }
        }
        n118 = call <vilib>:"Add State(s) to Queue__JKI_lib_State_Machine.vi"("State(s) in (\"\")"=w310) -> ("States Out"=w309:string)  [unwired: 14 in]
      }
      frame "UI: Front Panel State" {
        # "Argument"
        # "Set Front Panel Open or Closed\n(Usage: \"UI: Front Panel State >> Open|Close\")"
        n119 = Unbundle By Name(w318) -> ("Core.Current VI Reference"=w317:refnum<vi>)
        n120 = case shown="\"Minimize\", \"Minimized\"" w316 {
          tunnel: w320 -> [w328 w343 w354 w367 w380]
          tunnel: [w330 w344 w356 w369 w382] -> w319
          tunnel: w317 -> [w329 w341 w355 w368 w381]
          frame "Open", "Standard", Default {
            w323 = T1."Standard" ("State")
            n121 = property class="VI"(reference=w329, error in=w328) -> (reference out=w326:refnum<vi>, error out=w327:errorcluster, "FP.State"=w325:T1)
            n122 = Not Equal?(x=w325, y=w323) -> (x != y?=w324:bool)
            n123 = case shown="True" w324 {
              tunnel: [w334 w336] -> w330
              tunnel: w327 -> [w333 w336]
              tunnel: w326 -> [w332 _]
              tunnel: w323 -> [w331 _]
              frame True {
                n124 = invoke class="VI" method="FP.Open"(reference=w332, error in=w333, "Activate"=TRUE, "State"=w331) -> (error out=w334:errorcluster)  [unwired: 1 in, 4 out]
              }
              frame False {
              }
            }
          }
          frame "Close", "Closed" {
            n125 = property class="VI"(reference=w341, error in=w343) -> (reference out=w340:refnum<vi>, error out=w342:errorcluster, "FP.State"=w338:T1)
            n126 = Not Equal?(x=w338, y=T1."Closed" ("Front Panel Window:State")) -> (x != y?=w337:bool)
            n127 = case shown="True" w337 {
              tunnel: [w345 w348] -> w344
              tunnel: w342 -> [w345 w347]
              tunnel: w340 -> [_ w346]
              frame False {
              }
              frame True {
                n128 = invoke class="VI" method="FP.Close"(reference=w346, error in=w347) -> (error out=w348:errorcluster)  [unwired: 1 in, 2 out]
              }
            }
          }
          frame "Hidden", "Hide" {
            w349 = T1."Hidden" ("State")
            n129 = property class="VI"(reference=w355, error in=w354) -> (reference out=w352:refnum<vi>, error out=w353:errorcluster, "FP.State"=w351:T1)
            n130 = Not Equal?(x=w351, y=w349) -> (x != y?=w350:bool)
            n131 = case shown="True" w350 {
              tunnel: [w360 w361] -> w356
              tunnel: w353 -> [w359 w361]
              tunnel: w352 -> [w358 _]
              tunnel: w349 -> [w357 _]
              frame True {
                n132 = invoke class="VI" method="FP.Open"(reference=w358, error in=w359, "State"=w357) -> (error out=w360:errorcluster)  [unwired: 2 in, 4 out]
              }
              frame False {
              }
            }
          }
          frame "Minimize", "Minimized" {
            w362 = T1."Minimized" ("State")
            n133 = property class="VI"(reference=w368, error in=w367) -> (reference out=w365:refnum<vi>, error out=w366:errorcluster, "FP.State"=w364:T1)
            n134 = Not Equal?(x=w364, y=w362) -> (x != y?=w363:bool)
            n135 = case shown="True" w363 {
              tunnel: [w373 w374] -> w369
              tunnel: w366 -> [w372 w374]
              tunnel: w365 -> [w371 _]
              tunnel: w362 -> [w370 _]
              frame True {
                n136 = invoke class="VI" method="FP.Open"(reference=w371, error in=w372, "State"=w370) -> (error out=w373:errorcluster)  [unwired: 2 in, 4 out]
              }
              frame False {
              }
            }
          }
          frame "Maximize", "Maximized" {
            w375 = T1."Maximized" ("State")
            n137 = property class="VI"(reference=w381, error in=w380) -> (reference out=w378:refnum<vi>, error out=w379:errorcluster, "FP.State"=w377:T1)
            n138 = Not Equal?(x=w377, y=w375) -> (x != y?=w376:bool)
            n139 = case shown="True" w376 {
              tunnel: [w386 w387] -> w382
              tunnel: w379 -> [w385 w387]
              tunnel: w378 -> [w384 _]
              tunnel: w375 -> [w383 _]
              frame True {
                n140 = invoke class="VI" method="FP.Open"(reference=w384, error in=w385, "State"=w383) -> (error out=w386:errorcluster)  [unwired: 2 in, 4 out]
              }
              frame False {
              }
            }
          }
        }
        n141 = call <vilib>:"Add State(s) to Queue__JKI_lib_State_Machine.vi"("State(s) in (\"\")"=w322) -> ("States Out"=w321:string)  [unwired: 14 in]
      }
      frame "UI: Autoset Arguments" {
        n142 = call "CSM - Revert Arguments-Safe String.vi"("Safe Argurment String"=w399) -> ("Origin Argurment String"=w397:string)  [unwired: 8 in]
        n143 = control-ref of="CSM"() -> (w393:refnum<vi>)
        n144 = call "Remove Comments from Line.vi"("single-line text"=w397) -> ("single-line text without comments"=w398:string)  [unwired: 2 in]
        n145 = call "Splite Single-line Message.vi"("single-line text"=w398) -> ("state"=w395:string, "args"=w394:string, "source/target"=w390:string)  [unwired: 6 in, 1 out]
        n146 = property on="Property Node" class="CmbBox"(reference=w393) -> (reference out=w391:refnum<vi>, "Strings[]"=w392:string[])  [unwired: 1 in, 1 out]
        n147 = Search 1D Array(1D array=w392, element=w390) -> (index of element=w389:i32)  [unwired: 1 in]
        n148 = Greater Or Equal To 0?(x=w389) -> (x >= 0?=w388:bool)
        n149 = case shown="False" w388 {
          tunnel: w391 -> [_ w404]
          tunnel: w390 -> [_ w403]
          frame False {
          }
          frame True {
            n150 = property on="Property Node" class="CmbBox"(reference=w404, "Value"=w403) -> ()  [unwired: 1 in, 2 out]
          }
        }
        n151 = local write "Arguments"(w394) -> ()
        n152 = local write "CSM 2"(w395) -> ()
      }
      frame "UI: Refresh History List" {
        n153 = Unbundle By Name(w410) -> ("MessageList"=w406:string[])
        n154 = property on="History" class="LstBox (strict)"() -> ("Item Names"=w408:string[], "Value"=w409:i32)  [unwired: 2 in, 2 out]
        n155 = Index Array(array=w408, index=w409) -> (element=w407:string)
        n156 = Search 1D Array(1D array=w406, element=w407) -> (index of element=w405:i32)  [unwired: 1 in]
        n157 = property on="History" class="LstBox (strict)"("Item Names"=w406, "Value"=w405) -> ()  [unwired: 2 in, 2 out]
      }
      frame "UI: Refresh CSM List" {
        n158 = control-ref of="CSM"() -> (w422:refnum<vi>)
        n159 = property on="Property Node" class="CmbBox"(reference=w422) -> (reference out=w414:refnum<vi>, "Value"=w418:string)  [unwired: 1 in, 1 out]
        n160 = call "CSM - List Modules.vi"() -> ("Error out"=w421:errorcluster, "Module Names"=w416:string[])  [unwired: 10 in]
        n161 = Search 1D Array(1D array=w416, element=w418) -> (index of element=w420:i32)  [unwired: 1 in]
        n162 = Greater Or Equal To 0?(x=w420) -> (x >= 0?=w419:bool)
        n163 = Index Array(array=w416) -> (element=w417:string)  [unwired: 1 in]
        n164 = Select(t=w418, s=w419, f=w417) -> (s? t:f=w415:string)
        n165 = property on="Property Node" class="CmbBox"(reference=w414, "Strings[]"=w416, "Value"=w415) -> ()  [unwired: 1 in, 2 out]
        n166 = call <vilib>:"Simple Error Handler.vi"("error in (no error)"=w421) -> ()  [unwired: 4 in, 5 out]
      }
      frame "UI: Refresh UI" {
      }
      frame "---------- Macro ----------" {
        # "Do not put any code in this frame.\n(It is a separator no-op. You can make a copy of this frame to create a new Macro frame)"
        n167 = call <vilib>:"Add State(s) to Queue__JKI_lib_State_Machine.vi"("State(s) in (\"\")"=w435) -> ("States Out"=w434:string)  [unwired: 14 in]
      }
      frame "Macro: Initialize" {
        # "Initialization Macro\n(This is called once, when the VI starts)"
        n168 = call <vilib>:"Add State(s) to Queue__JKI_lib_State_Machine.vi"("State(s) in Front (\"\")"="Data: Initialize\nData: Initialize References\nInitialize Core Data\nEvents: Register\nUI: Initialize\nData: Load Arguments Config File\nUI: Front Panel State >> Open\nUI: Refresh CSM List\nUI: Refresh History List\nUI: Refresh UI", "State(s) in (\"\")"=w441) -> ("States Out"=w440:string)  [unwired: 13 in]
      }
      frame "Macro: Exit" {
        # "Exit Macro\n(This is called once, when the VI exits)"
        n169 = Unbundle By Name(w449) -> ("Core.Close Panel on Exit?"=w448:bool)
        n170 = Select(t="UI: Front Panel State >> Close", s=w448, f="") -> (s? t:f=w445:string)
        n171 = call <vilib>:"Add State(s) to Queue__JKI_lib_State_Machine.vi"("State(s) in (\"\")"=w445, "State(s) at Back (\"\")"="Data: Save Arguments Config File\nData: Cleanup\nEvents: Unregister\nExit") -> ("States Out"=w443:string)  [unwired: 13 in]
        n172 = call <vilib>:"Add State(s) to Queue__JKI_lib_State_Machine.vi"("State(s) in Front (\"\")"=w443, "State(s) in (\"\")"=w452) -> ("States Out"=w451:string)  [unwired: 13 in]
      }
      frame "---------- Action ----------" {
        # "Template Separator\n(You can make a copy of, or modify, this frame)"
        n173 = call <vilib>:"Add State(s) to Queue__JKI_lib_State_Machine.vi"("State(s) in (\"\")"=w457) -> ("States Out"=w456:string)  [unwired: 14 in]
      }
      frame "Action: Send CSM Message" {
        n174 = local read "CSM"() -> (w460:string)
        n175 = case shown="Default" "CSM 2" {
          selector: "CSM 2" -> [_ w473]
          tunnel: "Arguments" -> [_ w472]
          tunnel: [_ w478] -> w461
          tunnel: w460 -> [_ w471]
          tunnel: [_ w470] -> w459
          tunnel: "RespTMO(ms)" -> [_ w477]
          frame "" {
          }
          frame Default {
            n176 = call "CSM - Send Message and Wait for Reply.vi"("Response Timeout(5000ms)"=w477, "Current Module(\"\" to generate a ID)"="Tool-Testpnl" ("Current Module(\"\" to generate a ID)"), "Target Module"=w471, "Arguments (\"\")"=w472, "State"=w473) -> ("error out"=w478:errorcluster, "Response"=→"Response":string)  [unwired: 4 in, 1 out]
            n177 = call-poly "Build Message with Arguments++.vi"("State with Arguments"=w473, "Arguments (\"\")"=w472, "Target Module (\"\")"=w471) -> ("CSM Message String"=w475:string)  [unwired: 12 in]
            n178 = call "CSM - Make String Arguments Safe.vi"("Argurment String"=w475) -> ("Safe Argurment String"=w474:string)  [unwired: 8 in]
            n179 = call <vilib>:"Build State String with Arguments__JKI_lib_State_Machine.vi"("Arguments (\"\")"=w474, "State"="Data: Update Message List" ("State(s) in Front (\"\")")) -> ("State with Arguments"=w469:string)  [unwired: 4 in]
            n180 = call <vilib>:"Add State(s) to Queue__jki_lib_state_machine.vi"("State(s) in (\"\")"=w469, "State(s) at Back (\"\")"="UI: Refresh History List\nData: Save Arguments Config File" ("State(s) in Front (\"\")")) -> ("States Out"=w470:string)  [unwired: 13 in]
          }
        }
        n181 = call <vilib>:"Add State(s) to Queue__JKI_lib_State_Machine.vi"("State(s) in (\"\")"=w467, "State(s) at Back (\"\")"=w459) -> ("States Out"=w466:string)  [unwired: 13 in]
      }
      frame "Action: Post CSM Message" {
        # "Your code here.\n(You can make a copy of, or modify, this frame)"
        n182 = local read "Arguments"() -> (w482:string)
        n183 = local read "CSM 2"() -> (w481:string)
        n184 = local read "CSM"() -> (w484:string)
        n185 = case shown="Default" w481 {
          selector: w481 -> [_ w495]
          tunnel: w482 -> [_ w494]
          tunnel: [_ w499] -> w485
          tunnel: w484 -> [_ w493]
          tunnel: [_ w492] -> w483
          frame "" {
          }
          frame Default {
            n186 = call "CSM - Post Message.vi"("Current Module(\"\" to generate a ID)"="Tool-Testpnl" ("Current Module(\"\" to generate a ID)"), "Target Module"=w493, "Arguments (\"\")"=w494, "State"=w495) -> ("error out"=w499:errorcluster)  [unwired: 7 in]
            n187 = call-poly "Build Message with Arguments++.vi"("State with Arguments"=w495, "Arguments (\"\")"=w494, "Target Module (\"\")"=w493) -> ("CSM Message String"=w497:string)  [unwired: 12 in]
            n188 = call "CSM - Make String Arguments Safe.vi"("Argurment String"=w497) -> ("Safe Argurment String"=w496:string)  [unwired: 8 in]
            n189 = call <vilib>:"Build State String with Arguments__JKI_lib_State_Machine.vi"("Arguments (\"\")"=w496, "State"="Data: Update Message List" ("State(s) in Front (\"\")")) -> ("State with Arguments"=w491:string)  [unwired: 4 in]
            n190 = call <vilib>:"Add State(s) to Queue__JKI_lib_State_Machine.vi"("State(s) in (\"\")"=w491, "State(s) at Back (\"\")"="UI: Refresh History List\nData: Save Arguments Config File" ("State(s) in Front (\"\")")) -> ("States Out"=w492:string)  [unwired: 13 in]
          }
        }
        n191 = call <vilib>:"Add State(s) to Queue__JKI_lib_State_Machine.vi"("State(s) in (\"\")"=w489, "State(s) at Back (\"\")"=w483) -> ("States Out"=w488:string)  [unwired: 13 in]
      }
    }
  }
